vi "CSDB_Transfer.get instances&data from ini.vi"(4 "error in (no error)":errorcluster, 7 "configuration file path":path) -> (0 "error out":errorcluster, 2 "from ini data":string[][](array[string]), 3 "from ini instances":string[][](array[string]))   [LabVIEW 2014, in "CSDB_Transfer.lvlib"]
doc: "Reads all entries from an inifile."
uses:
  CSDB_Transfer.lvlib
  <vilib>/Utility/config.llb/Read Key (String).vi
  <vilib>/Utility/config.llb/NI_LVConfig.lvlib
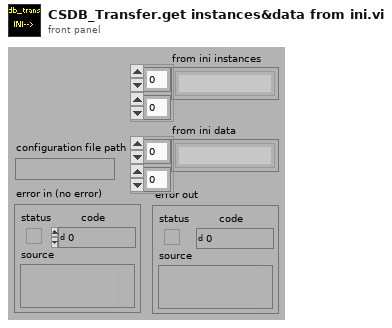
[diagram p1: front panel]
types:
  T1 = typedef "NI_LVConfig.lvlib/Config Data RefNum.ctl" = refnum<k1>
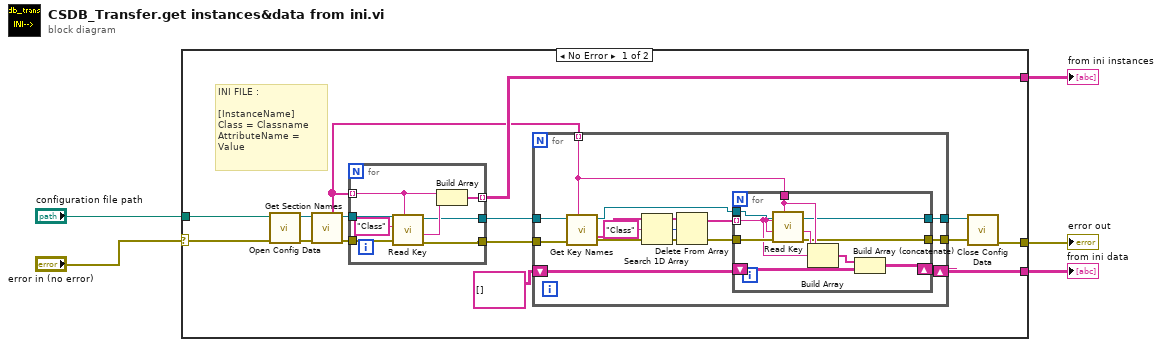
[diagram p0: block diagram]
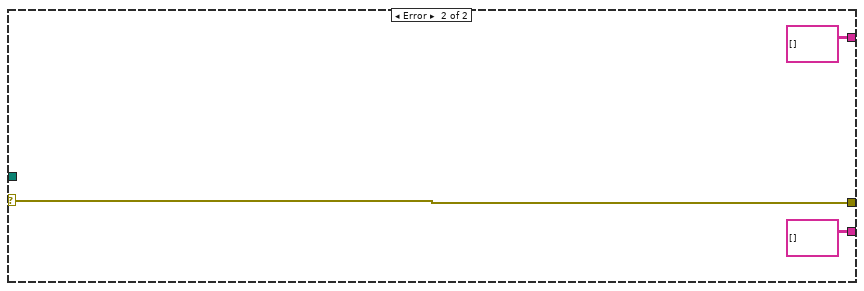
[diagram p2: hidden frame]
diagram:
  n1 = case shown="No Error" "error in (no error)" {
    selector: "error in (no error)" -> [w6 w54]
    tunnel: [w16 string[][] []] -> w5
    tunnel: [w15 w54] -> w4
    tunnel: [w8 string[][] []] -> w3
    tunnel: "configuration file path" -> [w7 _]
    frame No Error {
      # "INI FILE :\n\n[InstanceName]\nClass = Classname\nAttributeName = Value"
      n2 = call <vilib>:"Open Config Data.vi"("error in (no error)"=w6, "configuration file path"=w7) -> ("error out"=w19:errorcluster, "refnum"=w20:T1)  [unwired: 7 in, 1 out]
      n3 = call <vilib>:"Get Section Names.vi"("error in (no error)"=w19, "refnum"=w20) -> ("error out"=w17:errorcluster, "section names"=w14:string[], "refnum out"=w18:T1)  [unwired: 7 in]
      n4 = for {
        tunnel: w18 -> [w51]
        tunnel: w17 -> [w50]
        tunnel: w14 -> [w49] mode=indexing
        tunnel: [w46] -> w16 mode=indexing
        tunnel: [w45] -> w13
        tunnel: [w44] -> w12
        w47 = "Class" ("key")
        n5 = call-poly <vilib>:"Read Key.vi"("section"=w49, "error in (no error)"=w50, "default value"=w47, "key"=w47, "refnum"=w51) -> ("error out"=w44:errorcluster, "value"=w48:string, "refnum out"=w45:T1)  [unwired: 3 in, 1 out]
        n6 = Build Array(w49, w48) -> (w46:string[])
      }
      n7 = for {
        tunnel: w14 -> [w28] mode=indexing
        tunnel: w13 -> [w33]
        tunnel: w12 -> [w32]
        shift-right: [w24] -> w8
        shift-left: string[][] [] -> [w23]
        tunnel: [w22] -> w10
        tunnel: [w21] -> w9
        n8 = call <vilib>:"Get Key Names.vi"("section"=w28, "error in (no error)"=w32, "refnum"=w33) -> ("error out"=w26:errorcluster, "key names"=w29:string[], "refnum out"=w25:T1)  [unwired: 5 in, 1 out]
        n9 = Search 1D Array(1D array=w29, element="Class") -> (index of element=w30:i32)  [unwired: 1 in]
        n10 = Delete From Array(array=w29, index=w30) -> (array with subset deleted=w27:string[])  [unwired: 1 in, 1 out]
        n11 = for {
          tunnel: w28 -> [w41]
          tunnel: w27 -> [w40] mode=indexing
          tunnel: w26 -> [w43]
          tunnel: w25 -> [w42]
          shift-right: [w38] -> w24
          shift-left: w23 -> [w36]
          tunnel: [w35] -> w22
          tunnel: [w34] -> w21
          n12 = call-poly <vilib>:"Read Key.vi"("section"=w41, "error in (no error)"=w43, "default value"=w40, "key"=w40, "refnum"=w42) -> ("error out"=w34:errorcluster, "value"=w39:string, "refnum out"=w35:T1)  [unwired: 3 in, 1 out]
          n13 = Build Array(w41, w40, w39) -> (w37:string[])
          n14 = Build Array (concatenate)(w37, w36) -> (w38:string[][])
        }
      }
      n15 = call <vilib>:"Close Config Data.vi"("error in (no error)"=w9, "refnum"=w10) -> ("error out"=w15:errorcluster)  [unwired: 8 in, 1 out]
    }
    frame Error {
    }
  }
  "error out" <- w4
  "from ini instances" <- w5
  "from ini data" <- w3
